vi "Test Subtree.vi"() -> ()   [LabVIEW 2020, in "CDM-Config.lvlib"]
uses:
  CDM-Config.lvlib
  Config Manager/Config Manager.lvclass/Config Manager.ctl
  Config-JSON/Config-JSON.lvclass
  C:/dev/lv20CE/relink/lv-cdm/CDM-Config/Config Storage/Config Storage.lvclass
  Config Element/Set Owner.vi
  Config Element/Config Element.lvclass
  Config Storage/Config Storage.lvclass
  Config Manager/Config Manager.lvclass
panel:
  in  "Tree":string(tree)
  out "error out":errorcluster
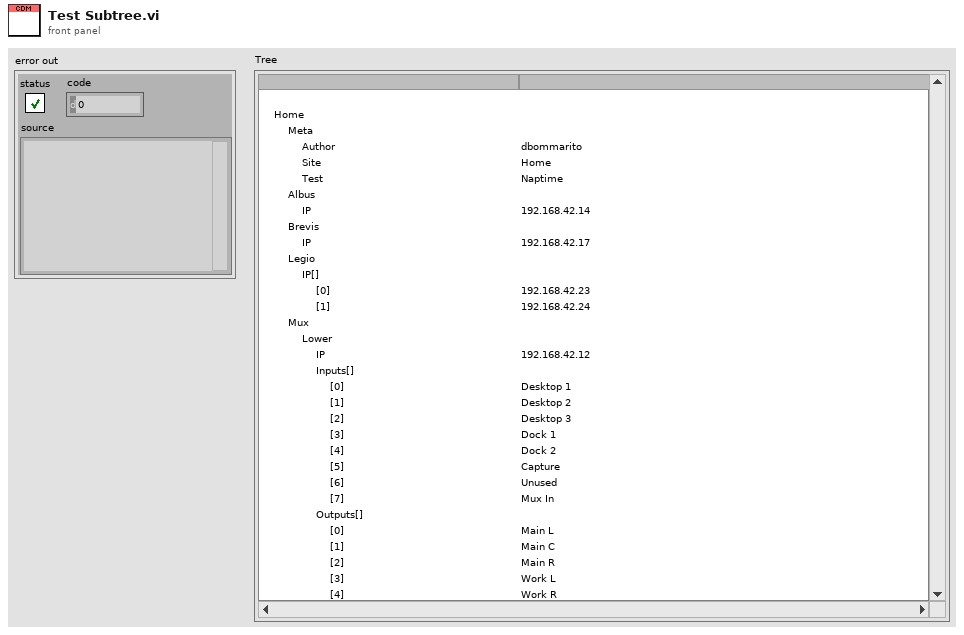
[diagram p1: front panel]
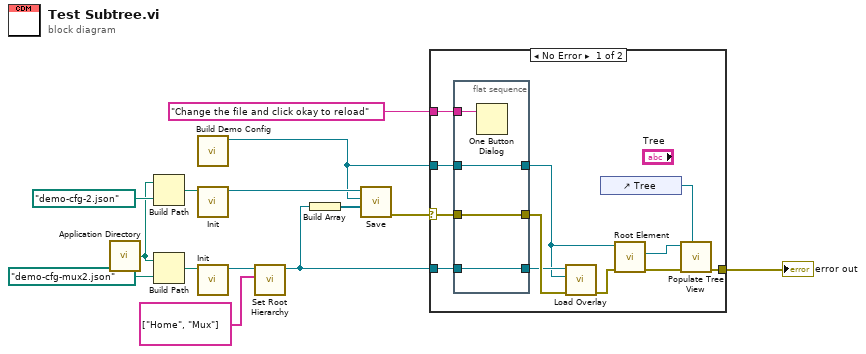
[diagram p0: block diagram]
diagram:
  n1 = call <vilib>:"Application Directory.vi"() -> ("Application Directory"=w8:path)
  n2 = Build Path(base path=w8, name or relative path=path "demo-cfg-2.json") -> (appended path=w10:path)
  n3 = Build Path(base path=w8, name or relative path=path "demo-cfg-mux2.json") -> (appended path=w13:path)
  n4 = call "Build Demo Config.vi"() -> ("Config Manager out"=w3:refnum<class "Config Manager.lvclass">)  [unwired: 11 in]
  n5 = call "Init.vi"("Path"=w10) -> ("Config-JSON out"=w7:refnum<class "Config-JSON.lvclass">)  [unwired: 9 in, 1 out]
  n6 = call "Init.vi"("Path"=w13) -> ("Config-JSON out"=w12:refnum<class "Config-JSON.lvclass">)  [unwired: 9 in, 1 out]
  n7 = call "Set Root Hierarchy.vi"("Root Hierarchy"=string[] ["Home", "Mux"], "Config Storage in"=w12) -> ("Config Storage out"=w2:refnum<class "Config-JSON.lvclass">)  [unwired: 8 in, 1 out]
  n8 = Build Array(w2) -> (w6:refnum<class "Config-JSON.lvclass">[])
  n9 = call "Save.vi"("Overlays (None)"=w6, "Config"=w3, "Config Storage in"=w7) -> ("error out"=w4:errorcluster)  [unwired: 7 in, 1 out]
  n10 = case shown="No Error" w4 {
    selector: w4 -> [w24 w31]
    tunnel: "Change the file and click okay to reload" ("message") -> [w25 _]
    tunnel: w3 -> [w23 _]
    tunnel: w2 -> [w22 _]
    tunnel: [w15 w31] -> w1
    frame No Error {
      n11 = flat-sequence {
        tunnel: w25 -> [w30]
        tunnel: w24 -> [w28]
        tunnel: w23 -> [w29]
        tunnel: [w29] -> w18
        tunnel: [w28] -> w26
        tunnel: w22 -> [w27]
        tunnel: [w27] -> w21
        frame #0 {
          n12 = One Button Dialog(message=w30) -> ()  [unwired: 1 in, 1 out]
        }
      }
      n13 = call "Load Overlay.vi"("error in (no error)"=w26, "Config"=w18, "Config Storage in"=w21) -> ("error out"=w19:errorcluster)  [unwired: 7 in, 1 out]
      n14 = control-ref of="Tree"() -> (w20:refnum<vi>)
      n15 = call "Root Element.vi"("error in (no error)"=w19, "Config Manager in"=w18) -> ("error out"=w17:errorcluster, "Root Element"=w16:refnum<class "Config Element.lvclass">)  [unwired: 7 in, 1 out]
      n16 = call "Populate Tree View.vi"("Tree"=w20, "error in (no error)"=w17, "Element"=w16) -> ("error out"=w15:errorcluster)  [unwired: 8 in]
    }
    frame Error {
    }
  }
  "error out" <- w1
